vi "error generator.vi"() -> ()   [LabVIEW 2020]
uses:
  Globals and TypeDefs/Error Categories.ctt
  <vilib>/Utility/error.llb/DialogType.ctl
panel:
  out "error out":errorcluster
  in  "error in (no error)":errorcluster
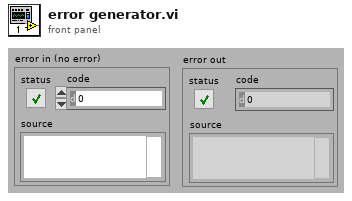
[diagram p1: front panel]
types:
  T1 = enum8{"Initialization Error", "Command Error", "Parameter Error", "Overflow Error", "Time-out Error", "Misc Error", "User cancel"}
  T2 = typedef "Error Categories.ctt" = enum8{"General", "CCD-256x1024", "CCD-1340x400", "InGaAs PDA", "McPherson 2075", "Magnetic Field", "Temperature Control", "Other"}
  T3 = typedef "DialogType.ctl" = u16
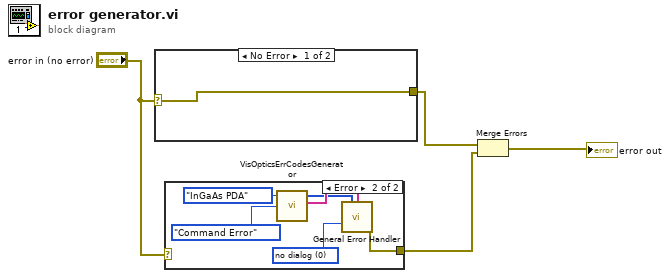
[diagram p0: block diagram]
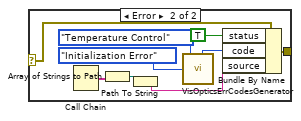
[diagram p3: hidden frame]
diagram:
  n1 = case shown="No Error" "error in (no error)" {
    selector: "error in (no error)" -> [w5 w6]
    tunnel: [w5 w12] -> w3
    frame No Error {
    }
    frame Error {
      n2 = Call Chain() -> (call chain=w9:string[])
      n3 = Array of Strings to Path(0:w9) -> (2:w8:path)  [unwired: 1 in]
      n4 = Path To String(path=w8) -> (string=w7:string)
      n5 = call "VisOpticsErrCodesGenerator.vi"("NHMFL Visible Optics Error Type"=T1."Initialization Error", "NHMFL Visible Optics Error Categories"=Error_Categories.ctt."Temperature Control") -> ("User-defined Error Code"=w10:i32)  [unwired: 1 in, 5 out]
      n6 = Bundle By Name(cluster=w6, "status"=TRUE, "code"=w10, "source"=w7) -> (w12:errorcluster)
    }
  }
  n7 = case shown="Error" "error in (no error)" {
    selector: "error in (no error)" -> [w15 _]
    tunnel: [w15 w16] -> w2
    frame No Error {
    }
    frame Error {
      w21 = T3 0 items=["no dialog", "OK message", "continue or stop message", "OK message + warnings", "continue/stop + warnings"] ("type of dialog (OK msg:1)")
      n8 = call "VisOpticsErrCodesGenerator.vi"("NHMFL Visible Optics Error Type"=T1."Command Error", "NHMFL Visible Optics Error Categories"=Error_Categories.ctt."InGaAs PDA") -> ("user-defined descriptions"=w20:string[], "user-defined codes"=w19:i32[])  [unwired: 1 in, 4 out]
      n9 = call <vilib>:"General Error Handler.vi"("[user-defined codes]"=w19, "[user-defined descriptions]"=w20, "type of dialog (OK msg:1)"=w21) -> ("error out"=w16:errorcluster)  [unwired: 8 in, 4 out]
    }
  }
  n10 = Merge Errors(w3, w2) -> (→"error out":errorcluster)
